vi "CheckPacket.vi"(8 "error in":errorcluster, 11 "Received":T1) -> (0 "error out":errorcluster)   [LabVIEW 2009]
uses:
  Packet.ctl
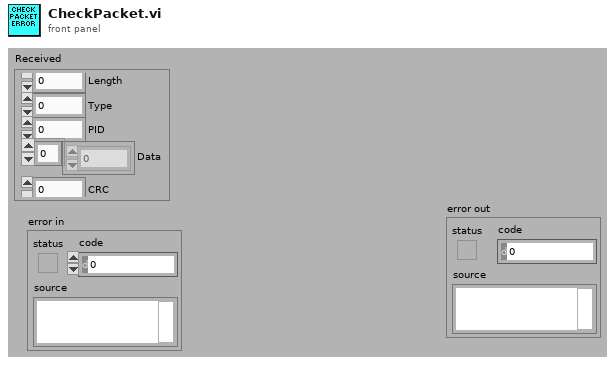
[diagram p1: front panel]
types:
  T1 = typedef "Packet.ctl" = cluster{"Length":u8, "Type":u8, "PID":u8, "Data":u8[], "CRC":u8}
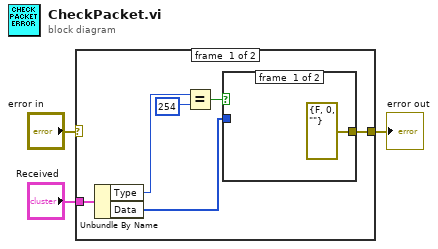
[diagram p0: block diagram]
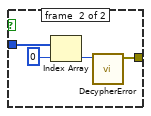
[diagram p2: hidden frame]
diagram:
  n1 = case shown="No Error" "error in" {
    selector: "error in" -> [_ w15]
    tunnel: [w6 w15] -> w2
    tunnel: "Received" -> [w9 _]
    frame #0 {
      n2 = Unbundle By Name(w9) -> ("Type"=w8:u8, "Data"=w4:u8[])
      n3 = Equal?(x=w8, y=u8 254) -> (x = y?=w5:bool)
      n4 = case shown="True" w5 {
        tunnel: [errorcluster {"status"=FALSE, "code"=0, "source"=""} ("error IO") w11] -> w6
        tunnel: w4 -> [_ w14]
        frame #0 {
        }
        frame #1 {
          n5 = Index Array(array=w14, index=0) -> (element=w12:u8)
          n6 = call "DecypherError.vi"("Numeric"=w12) -> ("error out"=w11:errorcluster)  [unwired: 10 in]
        }
      }
    }
    frame #1 {
    }
  }
  "error out" <- w2
